vi "Test XZ Single Ramp Approach Mode Waveforms.vi"() -> (0 "Reason":string, 1 "Success":bool)   [LabVIEW 2013]
uses:
  <vilib>/xml/Load XML File.vi
  <vilib>/xml/NI_XML.lvlib
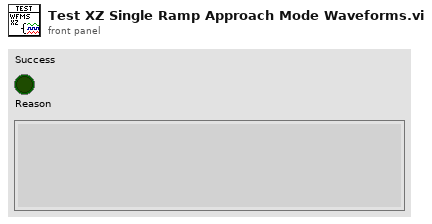
[diagram p1: front panel]
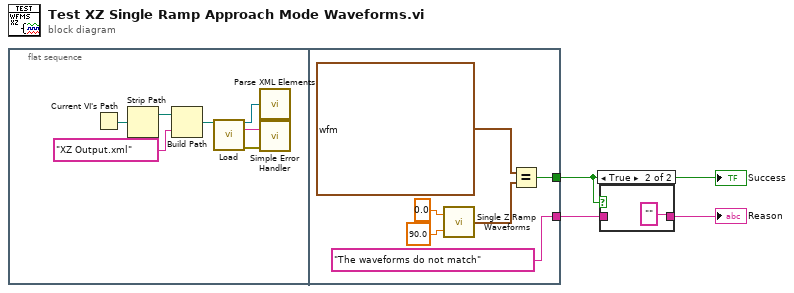
[diagram p0: block diagram]
diagram:
  n1 = flat-sequence {
    tunnel: [w14] -> w3
    tunnel: ["The waveforms do not match" ("name or relative path")] -> w1
    frame #0 {
      n2 = Current VI's Path() -> (path=w10:path)
      n3 = Strip Path(path=w10) -> (stripped path=w9:path)  [unwired: 1 out]
      n4 = Build Path(base path=w9, name or relative path="XZ Output.xml") -> (appended path=w4:path)
      n5 = call-poly <vilib>:"Load.vi"("path to XML document"=w4) -> ("DOM document out"=w7:refnum<k20>, "parse errors"=w5:string, "error out"=w6:errorcluster)  [unwired: 12 in]
      n6 = call "Parse XML Elements.vi"("DOM"=w7) -> ()
      n7 = call <vilib>:"Simple Error Handler.vi"("error source (\" \")"=w5, "error in (no error)"=w6) -> ()  [unwired: 3 in, 5 out]
    }
    frame #1 {
      n8 = call "Single Z Ramp Waveforms.vi"("Second Phase Offset"=90.0, "Initial Phase Offset"=0.0) -> ("Output Waveforms"=w12:waveform(dbl)[])
      n9 = Equal?(x=waveform(dbl)[] [{"t0"=timestamp(0 s since 1904-01-01), "dt"=0.0001, "Y"=array[10000 elements]}, {"t0"=timestamp(0 s since 1904-01-01), "dt"=0.0001, "Y"=array[10000 elements]}] ("Waveform Graph"), y=w12) -> (x = y?=w14:bool)
    }
  }
  n10 = case shown="True" w3 {
    tunnel: [w17 "" ("name or relative path")] -> w2
    tunnel: w1 -> [w17 _]
    frame False {
    }
    frame True {
    }
  }
  "Reason" <- w2
  "Success" <- w3
